vi "Tosca-Trace-Get Queue.vi"() -> (8 "Trace Queue":refnum<queue>, 15 "error out":errorcluster)   [LabVIEW 2020]
uses:
  Tosca-Trace Data.ctl
  Tosca-Trace-Event.ctl
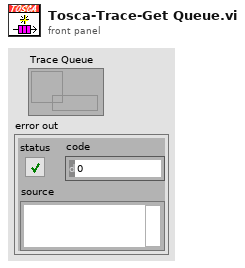
[diagram p1: front panel]
types:
  T1 = typedef "Tosca-Trace Data.ctl" = cluster{"Time":dbl, "Event":T2, "Source":string, "Message":string, "Data":dbl}
  T2 = typedef "Tosca-Trace-Event.ctl" = enum16{"Unspecified", "Trial start", "Enqueue", "Result", "End parser", "Frame", "Queue available", "Timeout sent", "WritePos", "TTL"}
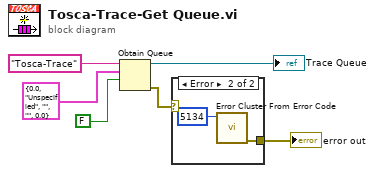
[diagram p0: block diagram]
diagram:
  n1 = Obtain Queue(name (unnamed)="Tosca-Trace", element data type=T1 {"Time"=0.0, "Event"=enum."Unspecified", "Source"="", "Message"="", "Data"=0.0} ("Trace Data"), create if not found? (T)=FALSE) -> (queue out=→"Trace Queue":refnum<queue>, error out=w2:errorcluster)  [unwired: 2 in, 1 out]
  n2 = case shown="Error" w2 {
    tunnel: [_ w8] -> w1
    frame No Error {
    }
    frame Error {
      n3 = call <vilib>:"Error Cluster From Error Code.vi"("error code (0)"=5134) -> ("error out"=w8:errorcluster)  [unwired: 8 in]
    }
  }
  "error out" <- w1
